vi "NI VeriStand FPGA RIO Library Example.vi"() -> ()   [LabVIEW 2009]
uses:
  <vilib>/Platform/TimedLoop/XDataNode/XDataNode.xnode
  <vilib>/Platform/TimedLoop/XDataNode/loadlvalarms.vi
  <vilib>/Platform/TimedLoop/XDataNode/timing_clust.ctl
  <vilib>/Platform/TimedLoop/XDataNode/nitl_modes.ctl
  <vilib>/Platform/TimedLoop/XDataNode/wakeup.ctl
  <userlib>/_NI VeriStand FPGA Support/NI VeriStand RIO Library/IP Based IO/Counter/common/CounterControl.ctl
  <vilib>/eio/EIONode/EIONode.xnode
  <vilib>/rvi/eio/nirviEIOImplementation/nirviEIOImplementation.xnode
  <vilib>/rvi/eio/common/nirviEmuTemplateMethod_noerrors.vi
  <vilib>/rvi/eio/common/nirviEmuClasses.ctl
  <vilib>/Platform/TimedLoop/XDataNode/XDNodeRunTimeDep.lvlib
  <vilib>/NI VeriStand/FPGA/NI_VS FPGA Support.lvlib
  <userlib>/_NI VeriStand FPGA Support/NI VeriStand FPGA Clock Support/NI_VS FPGA Clock Support.lvlib
panel:
  in  "PulseGen Packets":u64[](array[numeric])=[0, 0]
  out "Ctr Out":bool
  in  "Reset Counter":bool
  out "Counter Packet":u64
  in  "Ctr_Gate?":bool
  in  "Ctr_TickFilter":u32=2
  in  "Ctr_Edge":enum16{"Falling Edge", "Rising Edge"}(ring)=enum."Rising Edge"
  in  "Ctr_Cnt Dir":enum16{"Count Up", "Count Down"}(ring)
  in  "Ctr_Term Cnt":u64=16777216
  in  "Ctr_HiPulse":u32=1000
  out "Encoder Packets":u64[](array[numeric])
  in  "Encoder Interval (uSec)":u32=1000
  out "PulseMeas Packets":u64[](array[numeric])
  in  "PulseMeas 0 Timeout":u32=40000
  in  "PulseMeas 1 Timeout":u32=40000
  in  "PulseMeas 2 Timeout":u32=40000
  in  "PulseMeas 3 Timeout":u32=40000
  out "_PWM In Times":u64[](array[numeric])
  in  "_PWM Pulses 0-7":u64[](array[numeric])=[0, 0, 0, 0, 0, 0, 0, 0]
  in  "_PWM In 7 timeout":u32=40000
  in  "_PWM In 6 timeout":u32=40000
  in  "_PWM In 5 timeout":u32=40000
  in  "_PWM In 4 timeout":u32=40000
  in  "_PWM In 3 timeout":u32=40000
  in  "_PWM In 2 timeout":u32=40000
  in  "_PWM In 1 timeout":u32=40000
  in  "_PWM In 0 timeout":u32=40000
  in  "Generate IRQ":bool
  in  "Use External Timing":bool
  in  "Write to  RTSI":bool
  in  "Loop Rate (usec)":u32
  in  "Start":bool
  # "Counter"
  # "Pulse Generation"
  # "Encoder In"
  # "Pulse Measurement"
  # "PWM"
  # "Configuration"
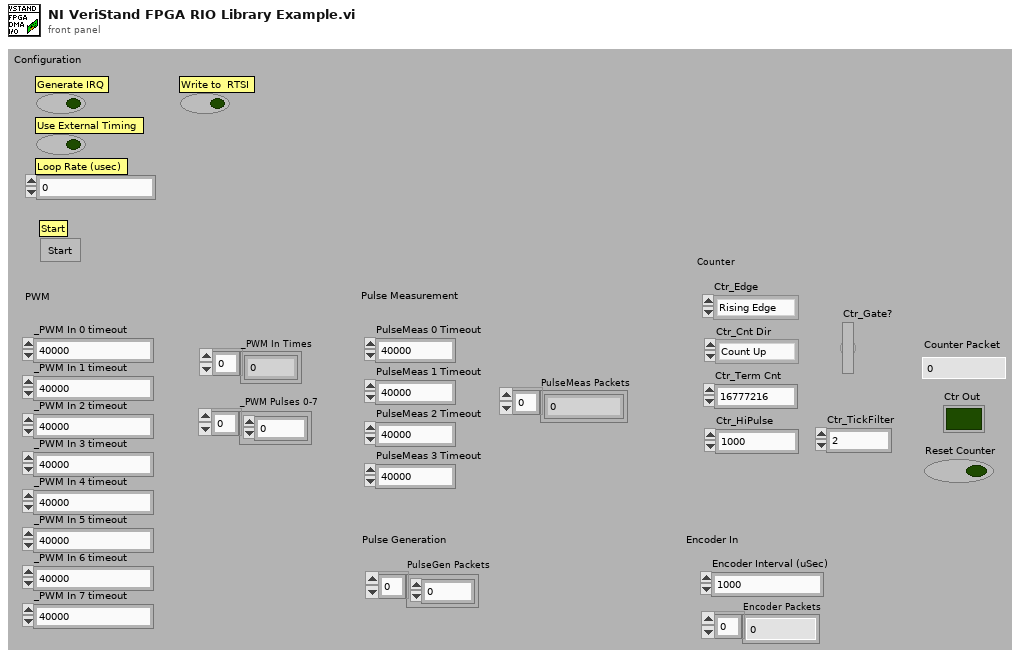
[diagram p1: front panel]
types:
  T1 = typedef "XDNodeRunTimeDep.lvlib/timing_clust.ctl" = cluster{"Expected End [f-1]":u64, "Actual End [f-1]":u64, "Finished Late? [f-1]":bool, "Expected End [i-1]":u64, "Actual End [i-1]":u64, "Finished Late? [i-1]":bool, "Expected Start [i]":u64, "Actual Start [i]":u64, "Expected Start [f]":u64, "Actual Start [f]":u64, "Source Name":string, "Structure Name":string, "Period":i64, "Deadline":i64, "Offset":i64, "Start":i64, "Priority":i32, "Timeout":i32, "Mode":T2, "Wakeup Reason":T3, "Error":errorcluster, "Source Type":string, "Secondary Source Type":string, "Global End Time":u64, "Global Start Time":u64, "Frame Duration":u64, "Iteration Duration":u64, "Assigned CPU":i32, "I/O Scan Engine Mode":u32}
  T2 = typedef "XDNodeRunTimeDep.lvlib/nitl_modes.ctl" = enum32{"No Change", "Process missed periods, maintain original phase", "Discard missed periods, maintain original phase", "Process missed periods, ignore original phase", "Discard missed periods, ignore original phase"}
  T3 = typedef "XDNodeRunTimeDep.lvlib/wakeup.ctl" = enum32{"Normal", "Aborted", "Asynchronous wakeup", "Timing source error", "Timed loop error", "Timeout"}
  T4 = cluster{"DO0":refnum<k21>, "DO1":refnum<k21>, "DO2":refnum<k21>, "DO3":refnum<k21>}
  T5 = cluster{"9263 AO0":refnum<k21>, "9263 AO1":refnum<k21>, "9263 AO2":refnum<k21>, "9263 AO3":refnum<k21>}
  T6 = cluster{"9215 AI0":refnum<k21>, "9215 AI1":refnum<k21>, "9215 AI2":refnum<k21>, "9215 AI3":refnum<k21>}
  T7 = typedef "CounterControl.ctl" = cluster{"Edge":enum16{"Falling Edge", "Rising Edge"}, "Gate?":bool, "Count Direction":enum16{"Count Up", "Count Down"}, "Terminal Count":u64, "Ticks to Filter":u32, "High Pulse Time (us)":u32}
  T8 = typedef "nirviEmuClasses.ctl" = enum16{"IO Read", "IO Write", "Method", "Property Read", "Property Write"}
  T9 = cluster{"DI0":refnum<k21>, "DI1":refnum<k21>, "DI2":refnum<k21>, "DI3":refnum<k21>, "DI4":refnum<k21>, "DI5":refnum<k21>, "DI6":refnum<k21>, "DI7":refnum<k21>}
  T10 = cluster{"DI0":refnum<k21>, "DI1":refnum<k21>, "DI2":refnum<k21>, "DI3":refnum<k21>}
  T11 = cluster{"DO0":refnum<k21>, "DO1":refnum<k21>, "DO2":refnum<k21>, "DO3":refnum<k21>, "DO4":refnum<k21>, "DO5":refnum<k21>, "DO6":refnum<k21>, "DO7":refnum<k21>}
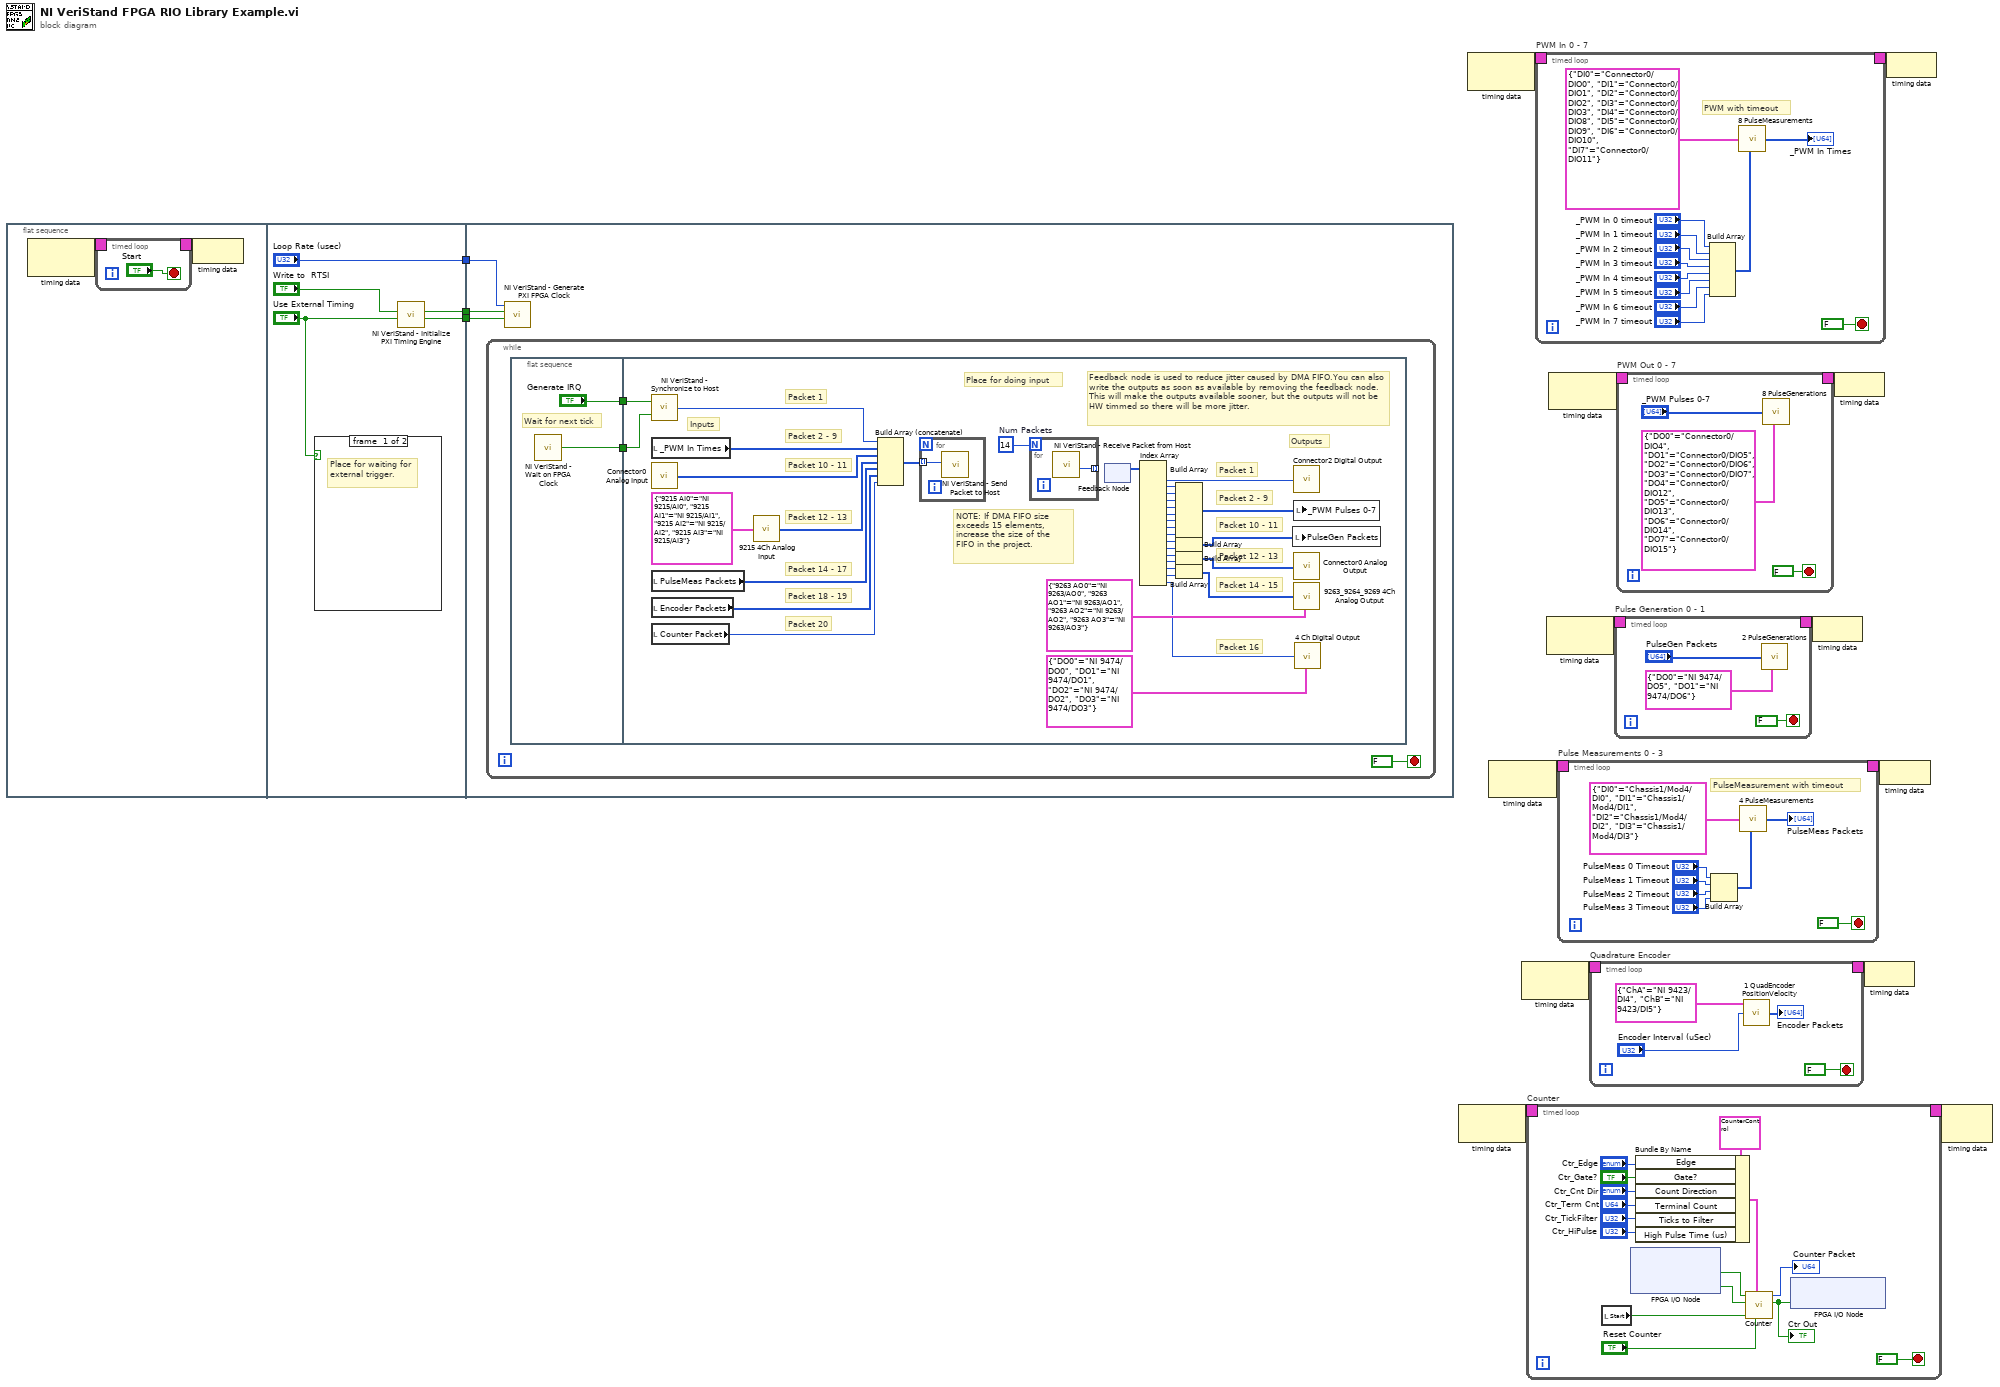
[diagram p0: block diagram]
diagram:
  n1 = flat-sequence {
    tunnel: [w24] -> w11
    tunnel: [w23] -> w10
    tunnel: ["Loop Rate (usec)"] -> w9
    tunnel: w11 -> [w30]
    tunnel: w10 -> [w29]
    tunnel: w9 -> [w28]
    frame #0 {
      n2 = node-c288() -> (w17:T1)  [unwired: 1 out]
      n3 = timed-loop {
        timing: w17 -> [_]
        timing-out: [_] -> w16
        stop <- "Start" stop-if-true
      }
      n4 = node-c288(w16) -> ()
    }
    frame #1 {
      n5 = case shown="False" "Use External Timing" {
        frame #0 {
          # "Place for waiting for external trigger."
        }
        frame #1 {
          # "Do not wait on trigger when externally timed."
        }
      }
      n6 = call <userlib>:"NI VeriStand - Initialize PXI Timing Engine.vi"("Use External Timing In"="Use External Timing", "Write to  RTSI In"="Write to  RTSI") -> ("Use External Timing Out"=w24:bool, "Write to  RTSI Out"=w23:bool)  [unwired: 8 in]
    }
    frame #2 {
      n7 = while {
        stop <- FALSE stop-if-true
        n8 = flat-sequence {
          tunnel: ["Generate IRQ"] -> w32
          tunnel: [w34] -> w31
          tunnel: w32 -> [w71]
          tunnel: w31 -> [w70]
          frame #0 {
            # "Wait for next tick"
            n9 = call <userlib>:"NI VeriStand - Wait on FPGA Clock.vi"() -> ("Clock Ticked"=w34:bool)
          }
          frame #1 {
            w69 = 14  # Num Packets
            # "Packet 14 - 15"
            # "Packet 20"
            # "Packet 18 - 19"
            # "Packet 14 - 17"
            # "Packet 16"
            # "Packet 12 - 13"
            # "Packet 12 - 13"
            # "Packet 1"
            # "Packet 10 - 11"
            # "Inputs"
            # "Outputs"
            # "Packet 2 - 9"
            # "Packet 10 - 11"
            # "Packet 2 - 9"
            # "Packet 1"
            # "NOTE: If DMA FIFO size exceeds 15 elements, increase the size of the FIFO in the project."
            # "Feedback node is used to reduce jitter caused by DMA FIFO.You can also write the outputs as soon as available by removing the feedback node.  This will make the outputs available sooner, but the outputs will not be HW timmed so there will be more jitter."
            # "Place for doing input"
            n10 = call <userlib>:"NI VeriStand - Synchronize to Host.vi"("Clock Ticked"=w70, "Generate IRQ"=w71) -> ("Is Late?"=w60:u64)
            n11 = local read "_PWM In Times"() -> (w59:u64[])
            n12 = call <userlib>:"Connector0 Analog Input.vi"() -> ("Packets"=w57:u64[])
            n13 = local read "PulseMeas Packets"() -> (w47:u64[])
            n14 = local read "Encoder Packets"() -> (w48:u64[])
            n15 = local read "Counter Packet"() -> (w46:u64)
            n16 = call <userlib>:"9215 4Ch Analog Input.vi"("9215 I/O"=T6 {"9215 AI0"="NI 9215/AI0", "9215 AI1"="NI 9215/AI1", "9215 AI2"="NI 9215/AI2", "9215 AI3"="NI 9215/AI3"}) -> ("Packets"=w56:u64[])
            n17 = Build Array (concatenate)(w60, w59, w57, w56, w47, w48, w46) -> (w58:u64[])
            n18 = for {
              tunnel: w58 -> [w72] mode=indexing
              n19 = call <vilib>:"NI VeriStand - Send Packet to Host.vi"("Element"=w72) -> ()  [unwired: 2 in, 9 out]
            }
            n20 = for {
              N: w69 -> [_]
              tunnel: [w73] -> w53 mode=indexing
              n21 = call <vilib>:"NI VeriStand - Receive Packet from Host.vi"() -> ("Element"=w73:u64)  [unwired: 2 in, 9 out]
            }
            n22 = feedback #1() -> (w52:u64[])  [unwired: 1 in]
            n23 = Index Array(array=w52) -> (element #1=w51:u64, element #2=w68:u64, element #3=w67:u64, element #4=w66:u64, element #5=w65:u64, element #6=w64:u64, element #7=w63:u64, element #8=w62:u64, element #9=w61:u64, element #10=w45:u64, element #11=w41:u64, element #12=w40:u64, element #13=w39:u64, element #14=w38:u64, element #15=w37:u64, element #16=w36:u64)  [unwired: 16 in]
            n24 = Build Array(w68, w67, w66, w65, w64, w63, w62, w61) -> (w50:u64[])
            n25 = Build Array(w45, w41) -> (w42:u64[])
            n26 = Build Array(w40, w39) -> (w44:u64[])
            n27 = Build Array(w38, w37) -> (w43:u64[])
            n28 = local write "PulseGen Packets"(w42) -> ()
            n29 = call <userlib>:"Connector2 Digital Output.vi"("Packet"=w51) -> ()
            n30 = local write "_PWM Pulses 0-7"(w50) -> ()
            n31 = call <userlib>:"Connector0 Analog Output.vi"("Packets"=w44) -> ()
            n32 = call <userlib>:"9263_9264_9269 4Ch Analog Output.vi"("Packets"=w43, "9263/4/9 I/O"=T5 {"9263 AO0"="NI 9263/AO0", "9263 AO1"="NI 9263/AO1", "9263 AO2"="NI 9263/AO2", "9263 AO3"="NI 9263/AO3"} ("9263 I/O")) -> ()  [unwired: 8 in]
            n33 = call <userlib>:"4 Ch Digital Output.vi"("Packet"=w36, "4 Ch Digital Out"=T4 {"DO0"="NI 9474/DO0", "DO1"="NI 9474/DO1", "DO2"="NI 9474/DO2", "DO3"="NI 9474/DO3"}) -> ()  [unwired: 8 in]
          }
        }
      }
      n34 = call <userlib>:"NI VeriStand - Generate PXI FPGA Clock.vi"("Use External Timing"=w30, "Write to  RTSI"=w29, "Loop Rate (usec)"=w28) -> ()  [unwired: 9 in]
    }
  }
  n35 = node-c288() -> (w4:T1)  [unwired: 1 in]
  n36 = node-c288() -> (w13:T1)  [unwired: 1 out]
  n37 = node-c288() -> (w6:T1)  [unwired: 1 out]
  n38 = node-c288() -> (w8:T1)  [unwired: 1 in]
  n39 = timed-loop "Counter" {
    timing: w4 -> [_]
    timing-out: [_] -> w3
    stop <- FALSE stop-if-true
    n40 = local read "Start"() -> (w74:bool)
    n41 = xnode "FPGA I/O Node"() -> ("NI 9423/DI6"=w84:bool, "NI 9423/DI7"=w85:bool)  [unwired: 2 in, 2 out]
    n42 = Bundle By Name(cluster=T7 {"Edge"=enum."Rising Edge", "Gate?"=TRUE, "Count Direction"=enum."Count Up", "Terminal Count"=16777216, "Ticks to Filter"=2, "High Pulse Time (us)"=1000} ("Counter Parameters"), "Edge"="Ctr_Edge", "Gate?"="Ctr_Gate?", "Count Direction"="Ctr_Cnt Dir", "Terminal Count"="Ctr_Term Cnt", "Ticks to Filter"="Ctr_TickFilter", "High Pulse Time (us)"="Ctr_HiPulse") -> (w81:T7)
    n43 = call <userlib>:"Counter.vi"("Reset Counter"="Reset Counter", "Counter Parameters"=w81, "Run?"=w74, "Ctr Gate"=w85, "Ctr Source"=w84) -> ("Ctr Out"=w83:bool, "Counter Register"=→"Counter Packet":u64)  [unwired: 5 in]
    "Ctr Out" <- w83
    n44 = xnode ("FPGA I/O Node")("NI 9474/DO4"=w83) -> ()  [unwired: 1 in, 1 out]
  }
  n45 = timed-loop "PWM In 0 - 7" {
    timing: w13 -> [_]
    timing-out: [_] -> w12
    stop <- FALSE stop-if-true
    # "PWM with timeout"
    n46 = Build Array("_PWM In 0 timeout", "_PWM In 1 timeout", "_PWM In 2 timeout", "_PWM In 3 timeout", "_PWM In 4 timeout", "_PWM In 5 timeout", "_PWM In 6 timeout", "_PWM In 7 timeout") -> (w141:u32[])
    n47 = call <userlib>:"8 PulseMeasurements.vi"("8 PulseMeas Chs"=T9 {"DI0"="Connector0/DIO0", "DI1"="Connector0/DIO1", "DI2"="Connector0/DIO2", "DI3"="Connector0/DIO3", "DI4"="Connector0/DIO8", "DI5"="Connector0/DIO9", "DI6"="Connector0/DIO10", "DI7"="Connector0/DIO11"} ("8 PWM In Chs"), "PulseMeas Timeouts"=w141) -> ("PulseMeas Packets"=→"_PWM In Times":u64[])  [unwired: 7 in]
  }
  n48 = node-c288() -> (w2:T1)  [unwired: 1 out]
  n49 = node-c288() -> (w15:T1)  [unwired: 1 out]
  n50 = timed-loop "Pulse Measurements 0 - 3" {
    timing: w6 -> [_]
    timing-out: [_] -> w5
    stop <- FALSE stop-if-true
    # "PulseMeasurement with timeout"
    n51 = Build Array("PulseMeas 0 Timeout", "PulseMeas 1 Timeout", "PulseMeas 2 Timeout", "PulseMeas 3 Timeout") -> (w160:u32[])
    n52 = call <userlib>:"4 PulseMeasurements.vi"("4 Pulse Meas Chs"=T10 {"DI0"="Chassis1/Mod4/DI0", "DI1"="Chassis1/Mod4/DI1", "DI2"="Chassis1/Mod4/DI2", "DI3"="Chassis1/Mod4/DI3"}, "PulseMeas Timeouts"=w160) -> ("PulseMeas Packets"=→"PulseMeas Packets":u64[])  [unwired: 7 in]
  }
  n53 = timed-loop "Quadrature Encoder" {
    timing: w8 -> [_]
    timing-out: [_] -> w7
    stop <- FALSE stop-if-true
    n54 = call <userlib>:"1 QuadEncoder PositionVelocity.vi"("Encoder Chs"=cluster{"ChA":refnum<k21>, "ChB":refnum<k21>} {"ChA"="NI 9423/DI4", "ChB"="NI 9423/DI5"}, "QuadEncoder Interval (uSec)"="Encoder Interval (uSec)") -> ("QuadEncoder Packets"=→"Encoder Packets":u64[])  [unwired: 7 in]
  }
  n55 = timed-loop "Pulse Generation 0 - 1" {
    timing: w2 -> [_]
    timing-out: [_] -> w1
    stop <- FALSE stop-if-true
    n56 = call <userlib>:"2 PulseGenerations.vi"("PulseGen Packets"="PulseGen Packets", "2 PulseGen Chs"=cluster{"DO0":refnum<k21>, "DO1":refnum<k21>} {"DO0"="NI 9474/DO5", "DO1"="NI 9474/DO6"}) -> ()  [unwired: 8 in]
  }
  n57 = timed-loop "PWM Out 0 - 7" {
    timing: w15 -> [_]
    timing-out: [_] -> w14
    stop <- FALSE stop-if-true
    n58 = call <userlib>:"8 PulseGenerations.vi"("PulseGen Packets"="_PWM Pulses 0-7", "8 PulseGen Chs"=T11 {"DO0"="Connector0/DIO4", "DO1"="Connector0/DIO5", "DO2"="Connector0/DIO6", "DO3"="Connector0/DIO7", "DO4"="Connector0/DIO12", "DO5"="Connector0/DIO13", "DO6"="Connector0/DIO14", "DO7"="Connector0/DIO15"} ("8 PWM Out Chs")) -> ()  [unwired: 8 in]
  }
  n59 = node-c288(w1) -> ()
  n60 = node-c288(w14) -> ()
  n61 = node-c288(w7) -> ()
  n62 = node-c288(w5) -> ()
  n63 = node-c288(w12) -> ()
  n64 = node-c288(w3) -> ()  [unwired: 1 out]
